vi "Get DataType.vi"(8 "error in (no error)":errorcluster, 11 "OD Entry in":refnum<class "OD Entry.lvclass">) -> (0 "error out":errorcluster, 2 "DataType":T1 items=["UNKNOWN", "BOOLEAN", "INTEGER8", "INTEGER16", "INTEGER32", "UNSIGNED8", "UNSIGNED16", "UNSIGNED32", "REAL32", "VISIBLE_STRING", "OCTET_STRING", "UNICODE_STRING", "TIME_OF_DAY", "TIME_DIFFERENCE", "DOMAIN", "INTEGER24", "REAL64", "INTEGER40", "INTEGER48", "INTEGER56", "INTEGER64", "UNSIGNED24", "UNSIGNED40", "UNSIGNED48", "UNSIGNED56", "UNSIGNED64", "PDO_COMMUNICATION_PARAMETER", "PDO_MAPPING", "SDO_PARAMETER", "IDENTITY"], 3 "OD Entry out":refnum<class "OD Entry.lvclass">)   [LabVIEW 2024, in "OD Entry.lvclass"]
uses:
  OD Entry.lvclass
  OD Entry.lvclass/OD Entry.ctl
  Data Type.ctl
  EDS.lvlib
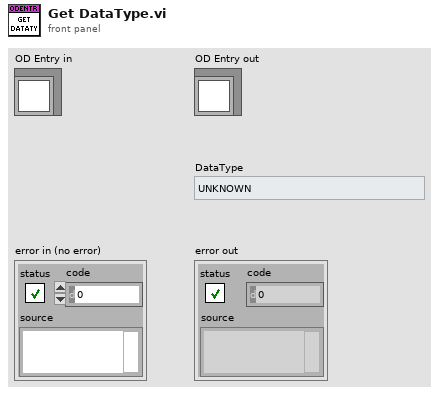
[diagram p1: front panel]
types:
  T1 = typedef "EDS.lvlib/Data Type.ctl" = u16
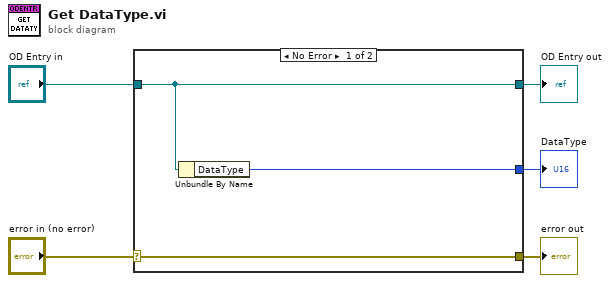
[diagram p0: block diagram]
diagram:
  n1 = case shown="No Error" "error in (no error)" {
    selector: "error in (no error)" -> [w8 w9]
    tunnel: [w8 w9] -> w4
    tunnel: [w7 w10] -> w2
    tunnel: "OD Entry in" -> [w7 w10]
    tunnel: [w6 _] -> w1
    frame No Error {
      n2 = Unbundle By Name(w7) -> ("DataType"=w6:T1)
    }
    frame Error {
    }
  }
  "error out" <- w4
  "OD Entry out" <- w2
  "DataType" <- w1
